vi "Close_Task.vi"(8 "error in (no error)":errorcluster caption="entrée d'erreur (pas d'erreur)", 11 "Class Log_File Altyor en entrée":refnum<class "Class Log_File Altyor.lvclass">) -> (0 "error out":errorcluster caption="sortie d'erreur", 3 "Class Log_File Altyor en sortie":refnum<class "Class Log_File Altyor.lvclass">)   [LabVIEW 2020, in "Library Instrument & Equipement.lvlib" / "Library Log_File.lvlib" / "Class Log_File Altyor.lvclass"]
uses:
  Class Log_File Altyor.lvclass
  Log_File (Default)/Class Log_File (Default).lvclass
  Class Log_File Altyor.lvclass/Class Log_File Altyor.ctl
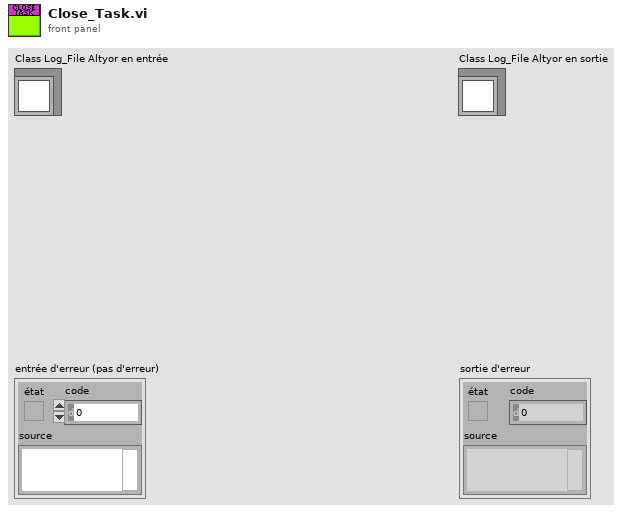
[diagram p1: front panel]
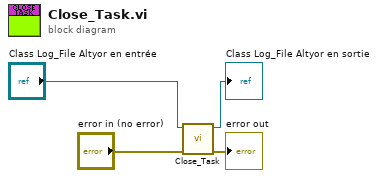
[diagram p0: block diagram]
diagram:
  n1 = call-parent "Close_Task.vi"("error in (no error)"="error in (no error)", "Class Log_File (Default) en entrée"="Class Log_File Altyor en entrée") -> ("error out"=→"error out":errorcluster, "Class Log_File (Default) en sortie"=→"Class Log_File Altyor en sortie":refnum<class "Class Log_File Altyor.lvclass">)  [unwired: 8 in]
